vi "senzorji.vi"() -> ()   [LabVIEW 2021]
panel:
  in  "bat 6":dbl
  in  "bat 5":dbl
  in  "bat 4":dbl
  in  "bat 3":dbl
  in  "bat 2":dbl
  in  "bat 1":dbl
  in  "Numeric 6":dbl
  in  "Numeric 5":dbl
  in  "Numeric 4":dbl
  in  "Numeric 3":dbl
  in  "Numeric 2":dbl
  in  "Numeric":dbl
  out "6":bool
  out "5":bool
  out "4":bool
  out "3":bool
  out "2":bool
  out "1":bool
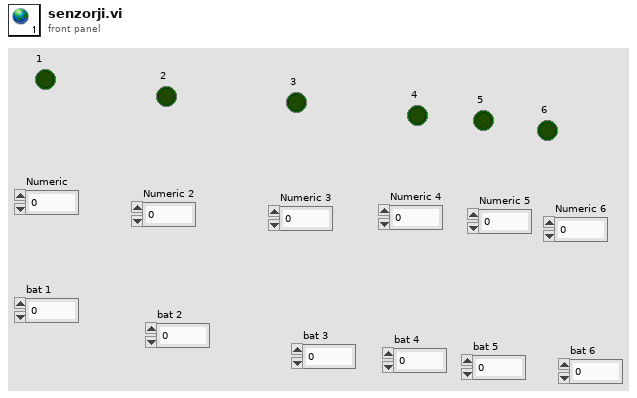
[diagram p1: front panel]
diagram:
